vi "Periodic Tasks.vi"(8 "error in":errorcluster) -> ()   [LabVIEW 2018]
doc: "This VI runs in parallel to other tasks. It can contain as many user-defined periodic loops as you need. These can carry out PID or other sorts of timed response."
uses:
  <vilib>/Rock Robotics/WPI/Utilities/WPI_GetSetVariantRefNum.vi
  <vilib>/Rock Robotics/Network Tables/NT Write Number.vi
panel:
  in  "FL Offset":dbl
  in  "FR Offset":dbl
  in  "BL Offset":dbl
  in  "BR Offset":dbl
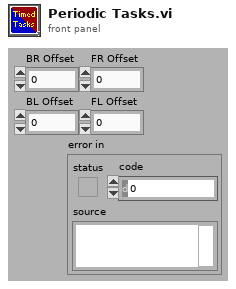
[diagram p1: front panel]
types:
  T1 = typedef "WPI_JoystickDevRef.ctl" = cluster{"Device":T2}
  T2 = typedef "WPI_JoystickDeviceEnum.ctl" = enum16{"USB 0", "USB 1", "USB 2", "USB 3", "USB 4", "USB 5"}
  T3 = typedef "WPI_AnalogChannelDevRef.ctl" = cluster{"DevStatus":errorcluster, "Analog Channel":T4}
  T4 = typedef "FPGA_AIChannel.ctl" = enum8{"AI 0", "AI 1", "AI 2", "AI 3", "AI MXP 0", "AI MXP 1", "AI MXP 2", "AI MXP 3", "Invalid"}
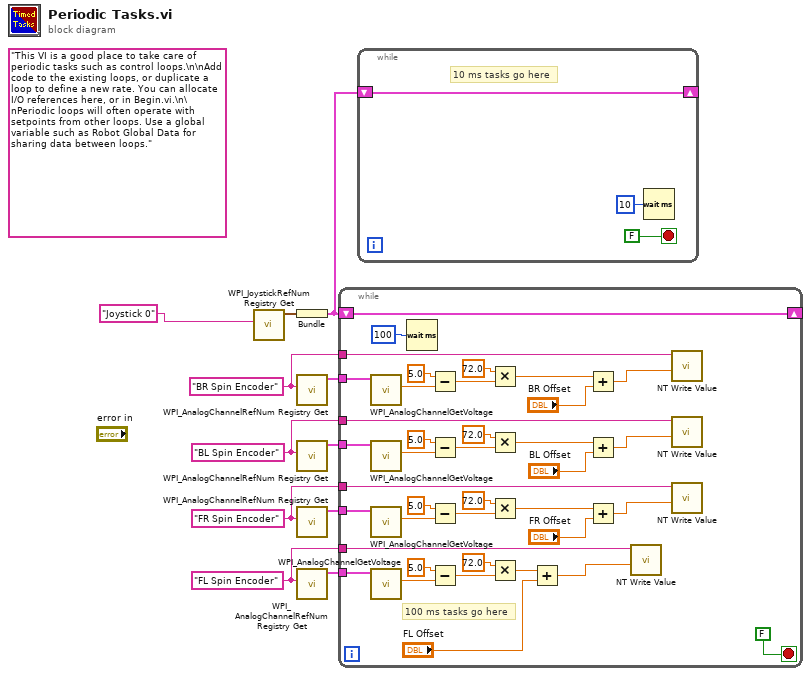
[diagram p0: block diagram]
diagram:
  w1 = "BR Spin Encoder" ("refnum name")
  w2 = "BL Spin Encoder" ("refnum name")
  w3 = "FR Spin Encoder" ("refnum name")
  w4 = "FL Spin Encoder" ("refnum name")
  (unwired) "This VI is a good place to take care of periodic tasks such as control loops.\n\nAdd code to the existing loops, or duplicate a loop to define a new rate. You can allocate I/O references here, or in Begin.vi.\n\nPeriodic loops will often operate with setpoints from other loops. Use a global variable such as Robot Global Data for sharing data between loops."
  n1 = call <vilib>:"WPI_JoystickRefNum Registry Get.vi"("refnum name"="Joystick 0") -> ("JoystickDevRef"=w10:T1)  [unwired: 1 in, 9 out]
  n2 = Bundle("JoystickDevRef"=w10) -> (w9:cluster{"JoystickDevRef":T1})  [unwired: 1 out]
  n3 = call <vilib>:"WPI_AnalogChannelRefNum Registry Get.vi"("refnum name"=w1) -> ("AIDeviceRef"=w5:T3)  [unwired: 9 in, 1 out]
  n4 = call <vilib>:"WPI_AnalogChannelRefNum Registry Get.vi"("refnum name"=w2) -> ("AIDeviceRef"=w6:T3)  [unwired: 9 in, 1 out]
  n5 = call <vilib>:"WPI_AnalogChannelRefNum Registry Get.vi"("refnum name"=w3) -> ("AIDeviceRef"=w7:T3)  [unwired: 9 in, 1 out]
  n6 = call <vilib>:"WPI_AnalogChannelRefNum Registry Get.vi"("refnum name"=w4) -> ("AIDeviceRef"=w8:T3)  [unwired: 9 in, 1 out]
  n7 = while {
    shift-right: [w48] -> _
    shift-left: w9 -> [w48]
    tunnel: w8 -> [w47]
    tunnel: w7 -> [w46]
    tunnel: w6 -> [w45]
    tunnel: w5 -> [w44]
    tunnel: w4 -> [w18]
    tunnel: w3 -> [w16]
    tunnel: w2 -> [w15]
    tunnel: w1 -> [w12]
    stop <- FALSE stop-if-true
    # "100 ms tasks go here"
    n8 = call <vilib>:"WPI_AnalogChannelGetVoltage.vi"("AIDeviceRef"=w44) -> ("Voltage"=w24:dbl)  [unwired: 8 in, 2 out]
    n9 = call <vilib>:"WPI_AnalogChannelGetVoltage.vi"("AIDeviceRef"=w45) -> ("Voltage"=w25:dbl)  [unwired: 8 in, 2 out]
    n10 = call <vilib>:"WPI_AnalogChannelGetVoltage.vi"("AIDeviceRef"=w46) -> ("Voltage"=w26:dbl)  [unwired: 8 in, 2 out]
    n11 = call <vilib>:"WPI_AnalogChannelGetVoltage.vi"("AIDeviceRef"=w47) -> ("Voltage"=w40:dbl)  [unwired: 8 in, 2 out]
    n12 = Wait (ms)(milliseconds to wait=u32 100) -> ()  [unwired: 1 out]
    n13 = Subtract(x=5.0, y=w24) -> (x-y=w30:dbl)
    n14 = Subtract(x=5.0, y=w25) -> (x-y=w31:dbl)
    n15 = Subtract(x=5.0, y=w26) -> (x-y=w38:dbl)
    n16 = Subtract(x=5.0, y=w40) -> (x-y=w39:dbl)
    n17 = Multiply(x=72.0 ("y"), y=w30) -> (x*y=w27:dbl)
    n18 = Multiply(x=72.0 ("y"), y=w31) -> (x*y=w34:dbl)
    n19 = Multiply(x=72.0 ("y"), y=w38) -> (x*y=w35:dbl)
    n20 = Multiply(x=72.0 ("y"), y=w39) -> (x*y=w43:dbl)
    n21 = Add(x=w43, y="FL Offset") -> (x+y=w19:dbl)
    n22 = Add(x=w27, y="BR Offset") -> (x+y=w13:dbl)
    n23 = Add(x=w34, y="BL Offset") -> (x+y=w14:dbl)
    n24 = Add(x=w35, y="FR Offset") -> (x+y=w17:dbl)
    n25 = call-poly <vilib>:"NT Write Value.vi"("Numeric"=w19, "Name"=w18) -> ()  [unwired: 9 in, 1 out]
    n26 = call-poly <vilib>:"NT Write Value.vi"("Numeric"=w13, "Name"=w12) -> ()  [unwired: 9 in, 1 out]
    n27 = call-poly <vilib>:"NT Write Value.vi"("Numeric"=w14, "Name"=w15) -> ()  [unwired: 9 in, 1 out]
    n28 = call-poly <vilib>:"NT Write Value.vi"("Numeric"=w17, "Name"=w16) -> ()  [unwired: 9 in, 1 out]
  }
  n29 = while {
    shift-right: [w51] -> _
    shift-left: w9 -> [w51]
    stop <- FALSE stop-if-true
    # "10 ms tasks go here"
    n30 = Wait (ms)(milliseconds to wait=u32 10) -> ()  [unwired: 1 out]
  }
